vi "Flatten.vi"(8 "error in (no error)":errorcluster, 11 "multimeter reader in":refnum<class "multimeter reader.lvclass">) -> (0 "error out":errorcluster, 3 "multimeter reader out":refnum<class "multimeter reader.lvclass">)   [LabVIEW 2017, in "multimeter reader.lvclass"]
uses:
  multimeter reader.lvclass
  multimeter reader.lvclass/multimeter reader.ctl
  Global/File Locations.vi
  Reader/Reader.lvclass
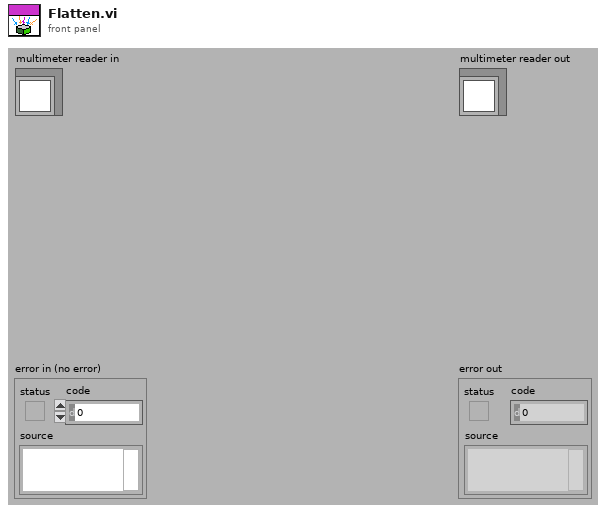
[diagram p1: front panel]
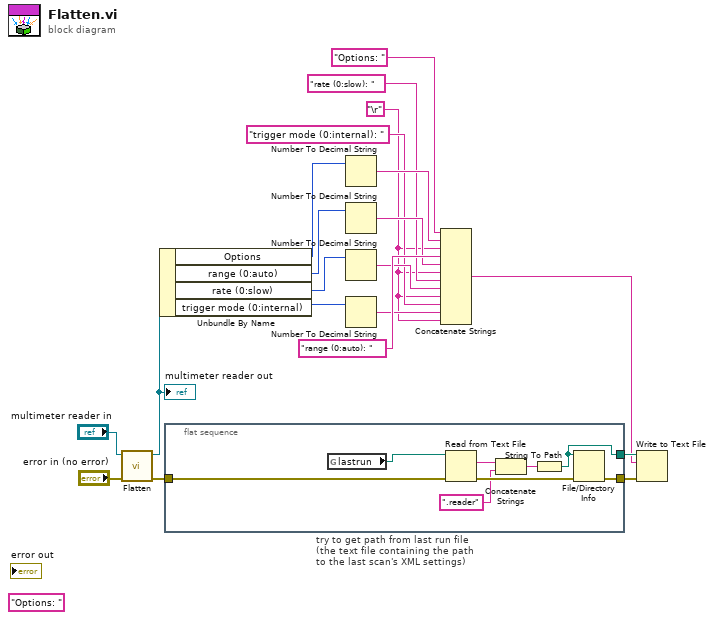
[diagram p0: block diagram]
diagram:
  (unwired) "Options: "
  w1 = "\r"
  n1 = call-parent "Flatten.vi"("error in (no error)"="error in (no error)", "Reader in"="multimeter reader in") -> ("error out"=w18:errorcluster, "Reader out"=w15:refnum<class "multimeter reader.lvclass">)  [unwired: 8 in]
  "multimeter reader out" <- w15
  n2 = Unbundle By Name(w15) -> ("Options"=w14:u16, "range (0:auto)"=w11:u16, "rate (0:slow)"=w12:u16, "trigger mode (0:internal)"=w13:u16)
  n3 = flat-sequence "try to get path from last run file\n(the text file containing the path\nto the last scan's XML settings)" {
    tunnel: [w28] -> w16
    tunnel: [w25] -> w17
    tunnel: w18 -> [w24]
    frame #0 {
      n4 = global read "File Locations.vi" "lastrun"() -> (w27:path)
      n5 = Read from Text File(file (use dialog)=w27, error in=w24) -> (text=w23:string, error out=w26:errorcluster)  [unwired: 4 out]
      n6 = Concatenate Strings(w23, ".reader") -> (w21:string)
      n7 = String To Path(string=w21) -> (path=w28:path)
      n8 = File/Directory Info(path=w28, error in=w26) -> (error out=w25:errorcluster)  [unwired: 6 out]
    }
  }
  n9 = Number To Decimal String(number=w14) -> (decimal integer string=w8:string)  [unwired: 1 in]
  n10 = Number To Decimal String(number=w11) -> (decimal integer string=w6:string)  [unwired: 1 in]
  n11 = Number To Decimal String(number=w12) -> (decimal integer string=w4:string)  [unwired: 1 in]
  n12 = Number To Decimal String(number=w13) -> (decimal integer string=w2:string)  [unwired: 1 in]
  n13 = Concatenate Strings("Options: ", w8, w1, "range (0:auto): ", w6, w1, "rate (0:slow): ", w4, w1, "trigger mode (0:internal): ", w2, w1) -> (w10:string)
  n14 = Write to Text File(file (use dialog)=w16, text=w10, error in=w17) -> ()  [unwired: 1 in, 3 out]
